vi "Inst_K2002.vi"(8 "error in":errorcluster, 10 "All Message Queues in":T1, 11 "Prueba31 in":refnum<class "Prueba04.lvclass">) -> (0 "error out":errorcluster)   [LabVIEW 2019, in "Prueba04.lvclass"]
uses:
  Prueba04.lvclass
  QMH/Message Queue/All Message Queues.ctl
  QMH/Message Queue/Message Cluster.ctl
  Prueba04.lvclass/Prueba04.ctl
  <vilib>/Utility/error.llb/Error Cluster From Error Code.vi
  QMH/Message Queue/Enqueue Message (Single).vi
  <vilib>/ErrorRing/Error Ring.xnode
  QMH/Message Queue/Message Queue.lvlib
  Instrumento/Keithley2002/Keithley2002.lvclass
panel:
  out "All States":string[](array[string])
  out "Actual State":string
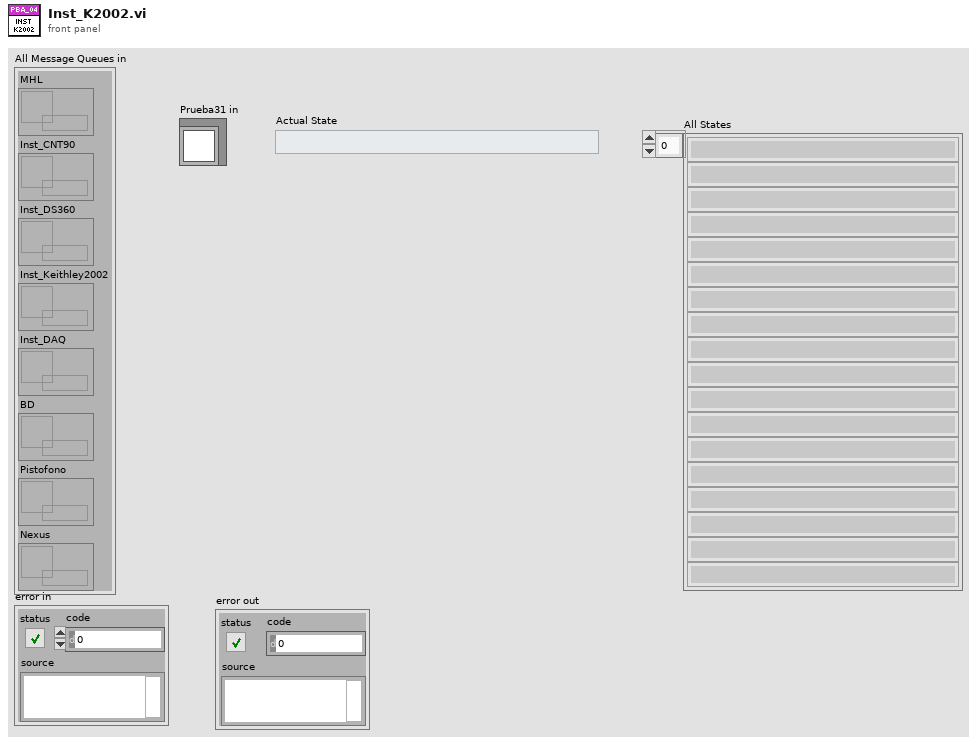
[diagram p1: front panel]
types:
  T1 = typedef "Message Queue.lvlib/All Message Queues.ctl" = cluster{"MHL":refnum<queue>, "Inst_CNT90":refnum<queue>, "Inst_DS360":refnum<queue>, "Inst_Keithley2002":refnum<queue>, "Inst_DAQ":refnum<queue>, "BD":refnum<queue>, "Pistofono":refnum<queue>, "Nexus":refnum<queue>}
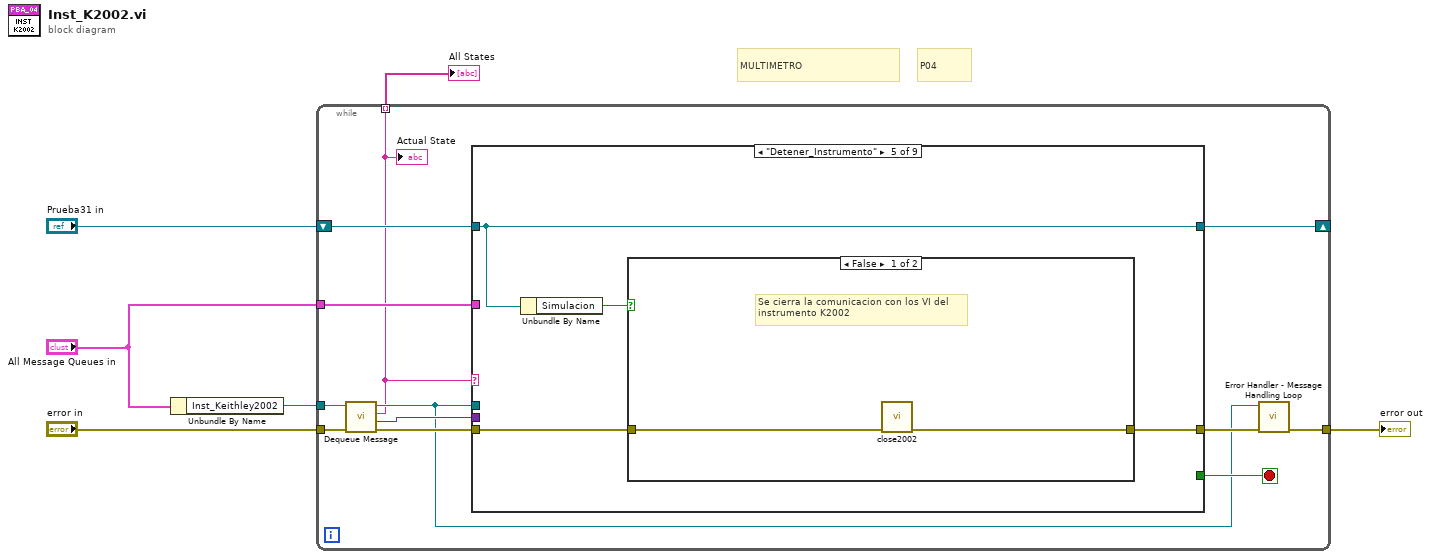
[diagram p0: block diagram]
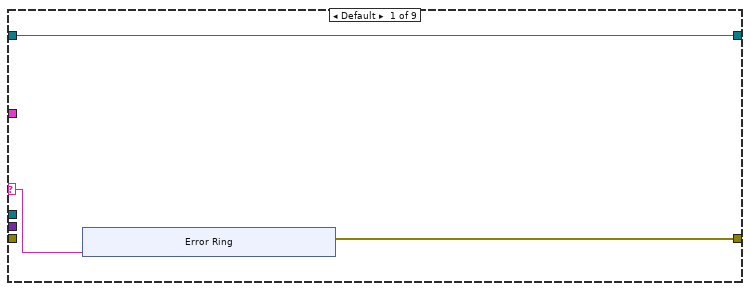
[diagram p2: hidden frame]
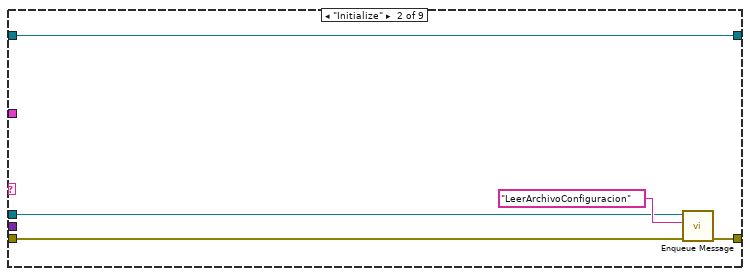
[diagram p3: hidden frame]
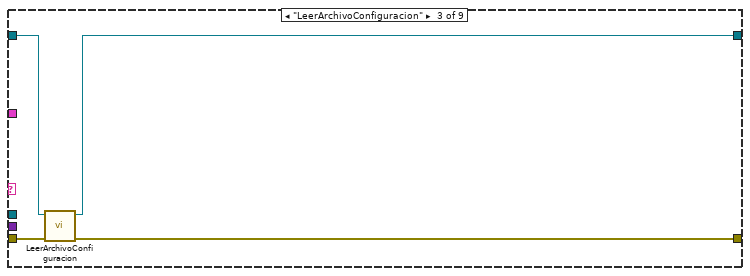
[diagram p4: hidden frame]
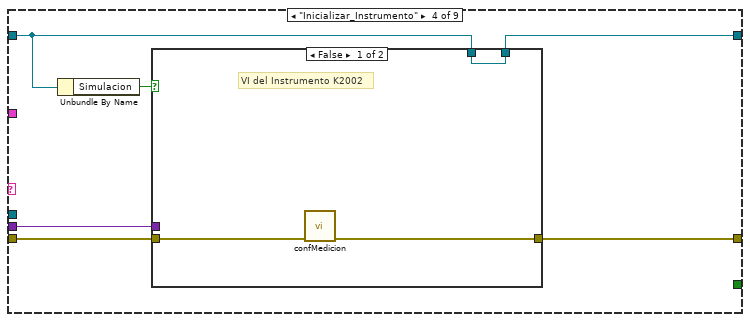
[diagram p5: hidden frame]
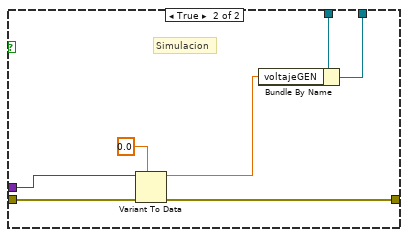
[diagram p6: hidden frame]
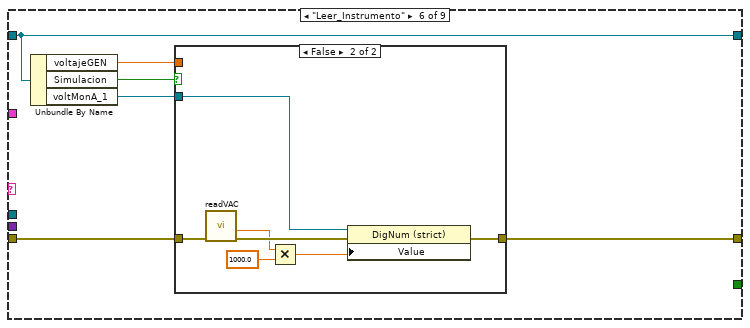
[diagram p8: hidden frame]
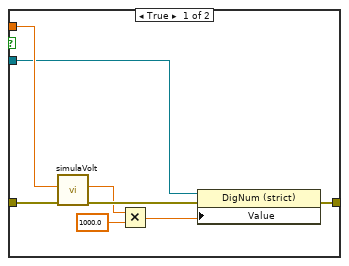
[diagram p9: hidden frame]
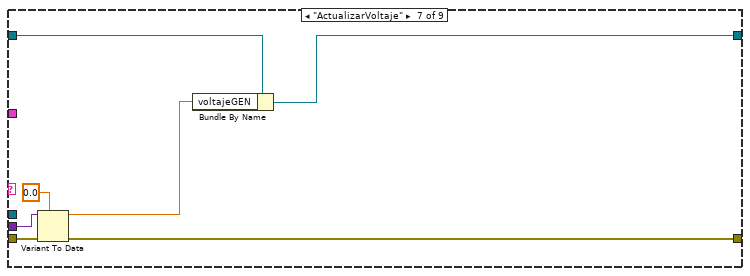
[diagram p10: hidden frame]
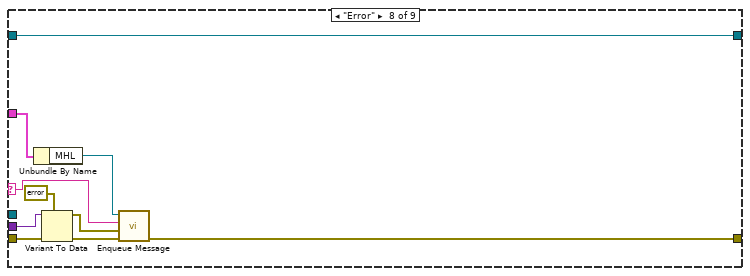
[diagram p11: hidden frame]
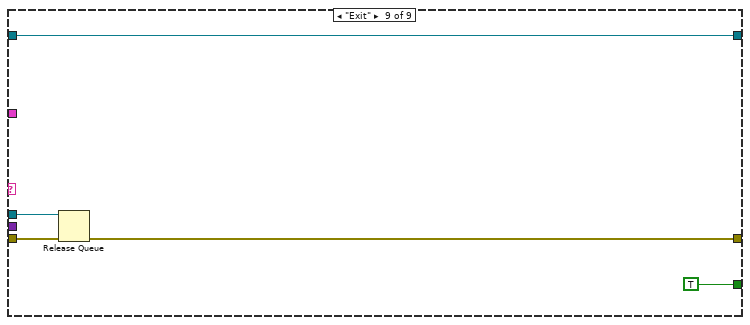
[diagram p12: hidden frame]
diagram:
  # "P04"
  # "MULTIMETRO"
  n1 = Unbundle By Name("All Message Queues in") -> ("Inst_Keithley2002"=w4:refnum<queue>)
  n2 = while {
    tunnel: "error in" -> [w18]
    tunnel: w4 -> [w17]
    tunnel: "All Message Queues in" -> [w16]
    tunnel: [w9] -> w2
    shift-right: [w12] -> _
    shift-left: "Prueba31 in" -> [w15]
    tunnel: [w7] -> w1 mode=indexing
    stop <- w11 stop-if-true
    n3 = call "Dequeue Message.vi"("error in (no error)"=w18, "Message Queue"=w17) -> ("error out"=w13:errorcluster, "Message Data"=w14:variant, "Message"=w7:string, "dup Message Queue"=w8:refnum<queue>)  [unwired: 6 in]
    "Actual State" <- w7
    n4 = case shown="\"Detener_Instrumento\"" w7 {
      selector: w7 -> [w21 _ _ _ _ _ _ w91 _]
      tunnel: w16 -> [_ _ _ _ _ _ _ w90 _]
      tunnel: w15 -> [w19 w33 w34 w40 w56 w66 w83 w98 w100]
      tunnel: w8 -> [_ w29 _ _ _ _ _ _ w102]
      tunnel: w14 -> [_ _ _ w38 _ _ w85 w95 _]
      tunnel: w13 -> [_ w31 w36 w41 w54 w64 w87 w96 w103]
      tunnel: [w20 w30 w37 w43 w57 w62 w88 w93 w99] -> w10
      tunnel: [w19 w33 w35 w39 w56 w66 w84 w98 w100] -> w12
      tunnel: [_ _ _ _ _ _ _ _ TRUE] -> w11
      frame Default {
        n5 = xnode "Error Ring"("parameter 0"=w21) -> ("error out"=w20:errorcluster)
      }
      frame "Initialize" {
        n6 = call-poly "Enqueue Message.vi"("error in (no error)"=w31, "Message"="LeerArchivoConfiguracion", "Message Queue"=w29) -> ("error out"=w30:errorcluster)  [unwired: 7 in, 1 out]
      }
      frame "LeerArchivoConfiguracion" {
        n7 = call "LeerArchivoConfiguracion.vi"("error in (no error)"=w36, "Prueba04 in"=w34) -> ("error out"=w37:errorcluster, "Prueba04 out"=w35:refnum<class "Prueba04.lvclass">)  [unwired: 8 in]
      }
      frame "Inicializar_Instrumento" {
        n8 = Unbundle By Name(w40) -> ("Simulacion"=w42:bool)
        n9 = case shown="False" w42 {
          tunnel: [w46 w50] -> w43
          tunnel: w41 -> [w45 w53]
          tunnel: w40 -> [w44 w52]
          tunnel: [w44 w51] -> w39
          tunnel: w38 -> [_ w49]
          frame False {
            # "VI del Instrumento K2002"
            n10 = call "confMedicion.vi"("error in (no error)"=w45) -> ("error out"=w46:errorcluster)  [unwired: 9 in, 1 out]
          }
          frame True {
            # "Simulacion"
            n11 = Variant To Data(error in=w53, type=0.0, Variant=w49) -> (data=w47:dbl, error out=w50:errorcluster)
            n12 = Bundle By Name(cluster=w52, "voltajeGEN"=w47) -> (w51:refnum<class "Prueba04.lvclass">)
          }
        }
      }
      frame "Detener_Instrumento" {
        n13 = Unbundle By Name(w56) -> ("Simulacion"=w55:bool)
        n14 = case shown="False" w55 {
          tunnel: [w59 w60] -> w57
          tunnel: w54 -> [w58 w60]
          frame False {
            # "Se cierra la comunicacion con los VI del\ninstrumento K2002"
            n15 = call "close2002.vi"("error in (no error)"=w58) -> ("error out"=w59:errorcluster)  [unwired: 9 in, 1 out]
          }
          frame True {
            # "Simulacion"
          }
        }
      }
      frame "Leer_Instrumento" {
        n16 = Unbundle By Name(w66) -> ("voltajeGEN"=w63:dbl, "Simulacion"=w65:bool, "voltMonA_1"=w61:refnum<vi>)
        n17 = case shown="False" w65 {
          tunnel: w64 -> [w74 w81]
          tunnel: w63 -> [w73 _]
          tunnel: [w69 w79] -> w62
          tunnel: w61 -> [w68 w78]
          frame True {
            n18 = call "simulaVolt.vi"("error in (no error)"=w74, "volt in"=w73) -> ("error out"=w70:errorcluster, "volt out"=w67:dbl)  [unwired: 7 in, 1 out]
            n19 = Multiply(x=w67, y=1000.0) -> (x*y=w71:dbl)
            n20 = property class="DigNum (strict)"(reference=w68, error in=w70, "Value"=w71) -> (error out=w69:errorcluster)  [unwired: 1 out]
          }
          frame False {
            n21 = call "readVAC.vi"("error in (no error)"=w81) -> ("error out"=w80:errorcluster, "medicion"=w77:dbl)  [unwired: 7 in, 2 out]
            n22 = Multiply(x=w77, y=1000.0) -> (x*y=w75:dbl)
            n23 = property class="DigNum (strict)"(reference=w78, error in=w80, "Value"=w75) -> (error out=w79:errorcluster)  [unwired: 1 out]
          }
        }
      }
      frame "ActualizarVoltaje" {
        n24 = Variant To Data(error in=w87, type=0.0, Variant=w85) -> (data=w82:dbl, error out=w88:errorcluster)
        n25 = Bundle By Name(cluster=w83, "voltajeGEN"=w82) -> (w84:refnum<class "Prueba04.lvclass">)
      }
      frame "Error" {
        n26 = Unbundle By Name(w90) -> ("MHL"=w89:refnum<queue>)
        n27 = Variant To Data(error in=w96, type=errorcluster {"status"=FALSE, "code"=0, "source"=""} ("error constant"), Variant=w95) -> (data=w92:errorcluster, error out=w94:errorcluster)
        n28 = call-poly "Enqueue Message.vi"("error in (no error)"=w94, "Message Data"=w92, "Message"=w91, "Message Queue"=w89) -> ("error out"=w93:errorcluster)  [unwired: 6 in, 1 out]
      }
      frame "Exit" {
        n29 = Release Queue(queue=w102, error in (no error)=w103) -> (error out=w99:errorcluster)  [unwired: 1 in, 2 out]
      }
    }
    n30 = call "Error Handler - Message Handling Loop.vi"("error in (no error)"=w10, "Message Queue"=w8) -> ("dup error in"=w9:errorcluster)  [unwired: 8 in, 1 out]
  }
  "error out" <- w2
  "All States" <- w1
